vi "cmd启动屏幕键盘.vi"(8 "error in (no error)":errorcluster caption="错误输入（无错误）", 11 "软键盘开关":enum16{"关闭", "打开"}(ring)) -> (0 "error out":errorcluster caption="错误输出", 2 "standard output":string caption="标准输出")   [LabVIEW 2017]
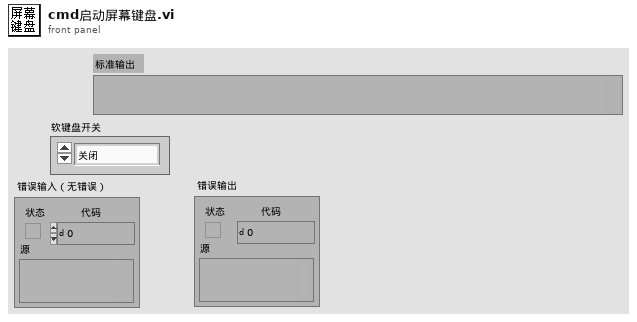
[diagram p1: front panel]
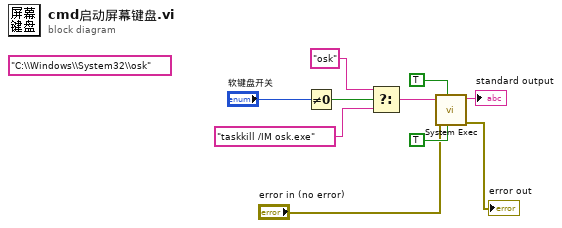
[diagram p0: block diagram]
diagram:
  (unwired) "C:\\Windows\\System32\\osk" ("command line")
  n1 = Not Equal To 0?(x="软键盘开关") -> (x != 0?=w7:bool)
  n2 = Select(t="osk" ("command line"), s=w7, f="taskkill /IM osk.exe" ("command line")) -> (s? t:f=w4:string)
  n3 = call <vilib>:"System Exec.vi"("run minimized? (F)"=TRUE, "wait until completion? (T)"=TRUE, "error in (no error)"="error in (no error)", "command line"=w4) -> ("error out"=→"error out":errorcluster, "standard output"=→"standard output":string)  [unwired: 4 in, 2 out]
